vi "Variant_To_DVR.vi"(8 "error in (no error)":errorcluster, 11 "Variant":variant) -> (0 "error out":errorcluster, 3 "DVR":refnum<data-value>)   [LabVIEW 2022 SP3, in "Motor Controller.lvclass"]
uses:
  Motor Controller.lvclass
  Typedefs/Private Data.ctl
  Typedefs/UserEvents.ctl
  Typedefs/API Event Data.ctl
  Typedefs/API Task State.ctl
  Typedefs/Status.ctl
  TopLevel/Typedefs/Motor Controller Config Data.ctl
  Typedefs/Stage Move Data.ctl
  Typedefs/Batch Index Speed Data.ctl
  Typedefs/Move Status.ctl
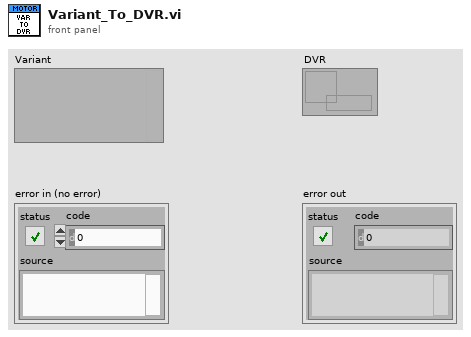
[diagram p1: front panel]
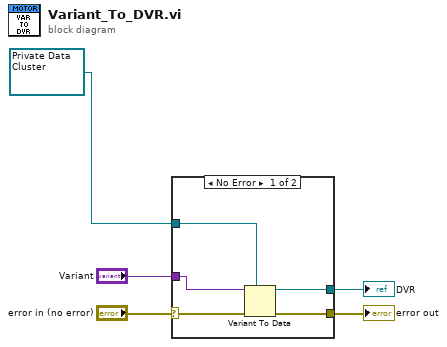
[diagram p0: block diagram]
diagram:
  n1 = case shown="No Error" "error in (no error)" {
    selector: "error in (no error)" -> [w10 w12]
    tunnel: [w9 w12] -> w4
    tunnel: "Variant" -> [w8 _]
    tunnel: [w7 w11] -> w1
    tunnel: refnum<data-value> refnum ("data value reference") -> [w6 w11]
    frame No Error {
      n2 = Variant To Data(error in=w10, type=w6, Variant=w8) -> (data=w7:refnum<data-value>, error out=w9:errorcluster)
    }
    frame Error {
    }
  }
  "error out" <- w4
  "DVR" <- w1
